vi "是否合法.vi"(8 "列":dbl, 9 "行":dbl, 11 "地图":dbl[][](array[numeric])) -> (2 "元素":dbl, 3 "是否合法":bool)   [LabVIEW 2012]
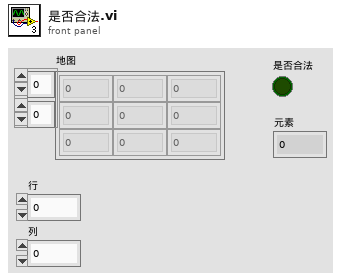
[diagram p1: front panel]
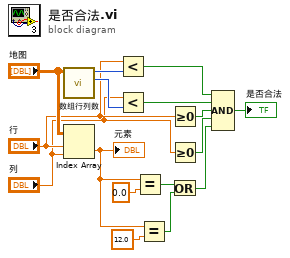
[diagram p0: block diagram]
diagram:
  n1 = call "数组行列数.vi"("数组"="地图") -> ("列"=w15:i32, "行"=w16:i32)  [unwired: 9 in]
  n2 = Index Array(array="地图", index (row)="行", index (col)="列") -> (element=w13:dbl)
  "元素" <- w13
  n3 = Less?(x="行", y=w16) -> (x < y?=w8:bool)
  n4 = Less?(x="列", y=w15) -> (x < y?=w7:bool)
  n5 = Equal?(x=w13, y=0.0) -> (x = y?=w9:bool)
  n6 = Equal?(x=w13, y=12.0) -> (x = y?=w10:bool)
  n7 = Greater Or Equal To 0?(x="行") -> (x >= 0?=w6:bool)
  n8 = Greater Or Equal To 0?(x="列") -> (x >= 0?=w5:bool)
  n9 = Or(x=w9, y=w10) -> (x .or. y?=w4:bool)
  n10 = Compound Arithmetic op=AND ("复合运算")(w8, w7, w6, w5, w4) -> (→"是否合法":bool)
